vi "Practica_1y2_Punto_3_1.vi"() -> ()   [LabVIEW 2020]
uses:
  <vilib>/numeric/Random Number (Range) U64.vi
  <vilib>/numeric/sub_Random U32.vi
panel:
  out "Waveform Chart":cluster{"number":u64, dbl, dbl}(graph)
  out "min value":dbl
  out "max value":dbl
  out "Filtro EMA":dbl[](array[numeric])
  out "Grados Celsius":dbl[](array[numeric])
  out "Grados Farenheit":dbl[](array[numeric])
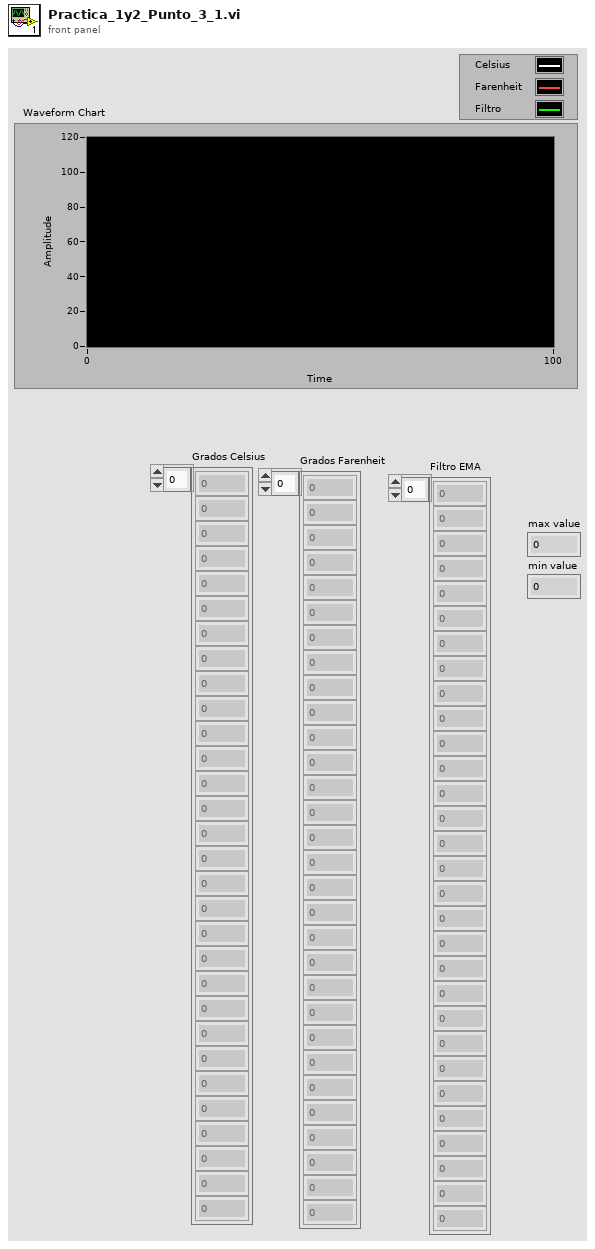
[diagram p1: front panel]
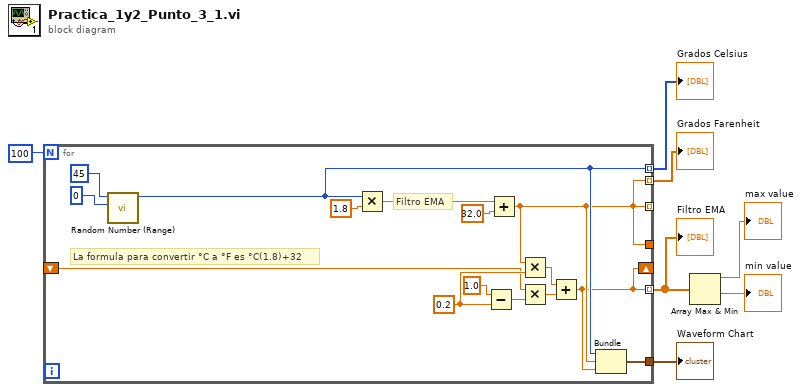
[diagram p0: block diagram]
diagram:
  n1 = for {
    N: 100 -> [_]
    tunnel: [w10] -> w2 mode=indexing
    tunnel: [w11] -> w4 mode=indexing
    tunnel: [w10] -> _ mode=indexing
    shift-right: [w9] -> _
    shift-left: _ -> [w12]
    tunnel: [w9] -> w3 mode=indexing
    tunnel: [w10] -> _
    tunnel: [w8] -> w1
    w15 = 0.2 ("y")
    # "Filtro EMA"
    # "La formula para convertir °C a °F es °C(1.8)+32"
    n2 = call-poly <vilib>:"Random Number (Range).vi"("lower bound (0)"=u64 0, "upper bound (100)"=u64 45) -> ("number"=w11:u64)  [unwired: 9 in]
    n3 = Multiply(x=w11, y=1.8) -> (x*y=w21:dbl)
    n4 = Subtract(x=1.0, y=w15) -> (x-y=w14:dbl)
    n5 = Add(x=w21, y=32.0) -> (x+y=w10:dbl)
    n6 = Multiply(x=w10, y=w15) -> (x*y=w17:dbl)
    n7 = Multiply(x=w12, y=w14) -> (x*y=w13:dbl)
    n8 = Add(x=w17, y=w13) -> (x+y=w9:dbl)
    n9 = Bundle("number"=w11, w10, w9) -> (w8:cluster{"number":u64, dbl, dbl})  [unwired: 1 in]
  }
  "Grados Farenheit" <- w2
  "Grados Celsius" <- w4
  "Filtro EMA" <- w3
  "Waveform Chart" <- w1
  n10 = Array Max & Min(array=w3) -> (max value=→"max value":dbl, min value=→"min value":dbl)  [unwired: 2 out]
